vi "Do.vi"(8 "error in (no error)":errorcluster, 10 "Actor in":refnum<class "Actor.lvclass">, 11 "Register Instrument Msg":refnum<class "Start Instrument Calibration Msg.lvclass">) -> (0 "error out":errorcluster, 2 "Actor out":refnum<class "Actor.lvclass">)   [LabVIEW 2020, in "Instrument Handler.lvlib" / "Start Instrument Calibration Msg.lvclass"]
doc: "This implementation sends itself to the Instrument Handler where it will start the calibration of all active instruments."
uses:
  Start Instrument Calibration Msg.lvclass
  C:/Current projects/WS/PPL/HDH.Actor Framework.Core.Actor.lvlibp/1abvi3w/vi.lib/ActorFramework/Message/Message.lvclass
  PPL/HDH.Actor Framework.Core.Actor.lvlibp/1abvi3w/vi.lib/ActorFramework/Actor/Actor.lvclass
  Instrument Handler/Instrument Handler.lvclass
  C:/Current projects/WS/PPL/HDH.Actor Framework.Core.Actor.lvlibp/1abvi3w/vi.lib/ActorFramework/Actor/Actor.lvclass
  PPL/HDH.Actor Framework.Core.Publisher.lvlibp/Publisher Messages/Targetted Msg/Targetted Msg.lvclass
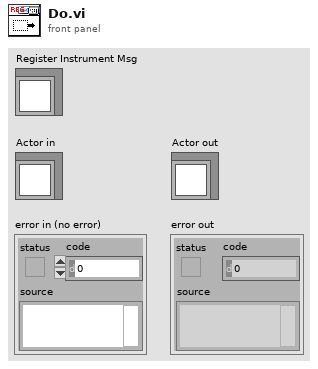
[diagram p1: front panel]
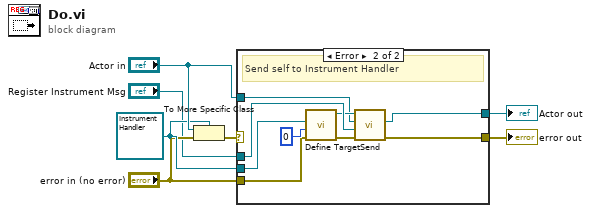
[diagram p0: block diagram]
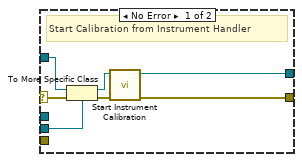
[diagram p2: hidden frame]
diagram:
  w3 = refnum<class "Instrument Handler.lvclass"> refnum ("Actor in")
  n1 = To More Specific Class(target class=w3, reference="Actor in", error in="error in (no error)") -> (error out=w7:errorcluster)  [unwired: 1 out]
  n2 = case shown="Error" w7 {
    selector: w7 -> [w12 _]
    tunnel: [w8 w15] -> w6
    tunnel: [w10 w17] -> w5
    tunnel: "Actor in" -> [w14 w18]
    tunnel: w3 -> [w13 w23]
    tunnel: "error in (no error)" -> [_ w21]
    tunnel: "Register Instrument Msg" -> [_ w20]
    frame No Error {
      # "Start Calibration from Instrument Handler"
      n3 = To More Specific Class(target class=w13, reference=w14, error in=w12) -> (specific class reference=w11:refnum<class "Instrument Handler.lvclass">, error out=w9:errorcluster)
      n4 = call "Start Instrument Calibration.vi"("error in (no error)"=w9, "Instrument Handler in"=w11) -> ("error out"=w8:errorcluster, "Instrument Handler out"=w10:refnum<class "Instrument Handler.lvclass">)  [unwired: 8 in]
    }
    frame Error {
      # "Send self to Instrument Handler"
      n5 = call "Define Target.vi"("error in (no error)"=w21, "Target Actor index(-1, all)"=0, "Target Actor"=w23) -> ("error out"=w16:errorcluster, "Targetted Msg out"=w19:refnum<class "Targetted Msg.lvclass">)  [unwired: 7 in]
      n6 = call-dynamic "Send.vi"("error in (no error)"=w16, "Message"=w20, "Actor in"=w18, "Targetted Msg in"=w19) -> ("error out"=w15:errorcluster, "Actor out"=w17:refnum<class "Actor.lvclass">)  [unwired: 5 in, 1 out]
    }
  }
  "error out" <- w6
  "Actor out" <- w5
